vi "Check 3765 Card Exist.vi"(8 "error in (no error)":errorcluster) -> (0 "error out":errorcluster, 2 "Boolean":bool)   [LabVIEW 2016, in "Hall Effect Library.lvlib"]
uses:
  Hall Effect Library.lvlib
  Global Variables/Instruments.vi
  Global Variables/Test Settings.vi
  Global Variables/Instrument Locations.vi
  <instrlib>/Keithley 3706/Keithley 3706.lvlib
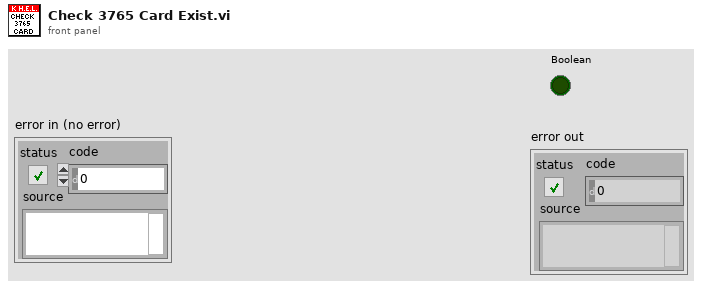
[diagram p1: front panel]
types:
  T1 = typedef "Hall Effect Library.lvlib/Switches.ctl" = enum16{"3706A"}
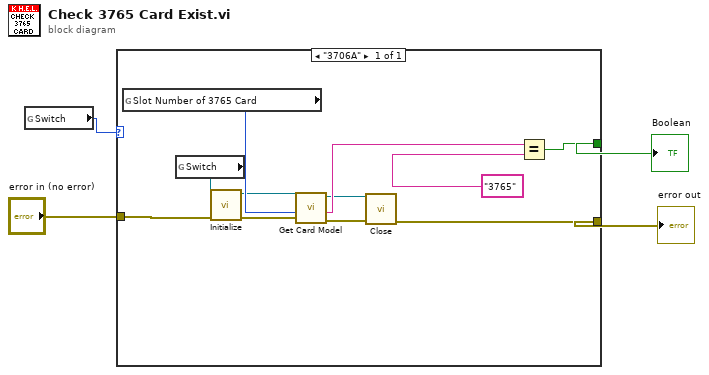
[diagram p0: block diagram]
diagram:
  n1 = global read "Instruments.vi" "Switch"() -> (w4:T1)
  n2 = case shown="\"3706A\"" w4 {
    tunnel: "error in (no error)" -> [w10]
    tunnel: [w5] -> w2
    tunnel: [w12] -> w1
    frame "3706A" {
      n3 = global read "Test Settings.vi" "Slot Number of 3765 Card"() -> (w15:u32)
      n4 = global read "Instrument Locations.vi" "Switch"() -> (w11:refnum<visa-resource-name>)
      n5 = call <instrlib>:"Initialize.vi"("error in (no error)"=w10, "VISA resource name"=w11) -> ("error out"=w8:errorcluster, "VISA resource name out"=w9:refnum<visa-resource-name>)  [unwired: 8 in]
      n6 = call <instrlib>:"Get Card Model.vi"("error in (no error)"=w8, "Slot Number"=w15, "VISA resource name"=w9) -> ("error out"=w7:errorcluster, "Card Model"=w13:string, "VISA resource name out"=w6:refnum<visa-resource-name>)  [unwired: 6 in]
      n7 = call <instrlib>:"Close.vi"("error in (no error)"=w7, "VISA resource name"=w6) -> ("error out"=w5:errorcluster)  [unwired: 9 in]
      n8 = Equal?(x=w13, y="3765") -> (x = y?=w12:bool)
    }
  }
  "error out" <- w2
  "Boolean" <- w1
